vi "control loop output action.vi"(11 "control loop data in":T1) -> (3 "control loop data out":T1)   [LabVIEW 2013, in "main engine.lvlib"]
doc: "This VI calls the output method of any modules specified by flags set in 'engine schedule.module run flags'. It also exchanges the data necessary for that method with the data in the engine tag bus. Any errors that occur are stored to be handled at the end of the engine's execution.\n\nSynchronous calls are handled inline. Asynchronous calls use a FIFO to communicate with a separate process launched during the initialization process."
uses:
  main engine.lvlib
  control loop data.ctl
  <vilib>/NI/Tag Bus/table/data table.ctl
  engine run schedule.ctl
  engine decimation schedule.ctl
  full module data.ctl
  <vilib>/NI/Tag Bus Module Framework/runtime/TBM module execution interface.lvclass
  module run state.ctl
  async executor/asynchronous executor reference.ctl
  async executor/async message to executor.ctl
  Runtime/async command notification.ctl
  Runtime/async error info.ctl
  <vilib>/NI/Tag Bus Module Framework/runtime/error classification.ctl
  <vilib>/NI/Tag Bus Module Framework/module configuration/TBM module configuration.lvclass
  module method data.ctl
  <vilib>/NI/Tag Bus/table/transfer specification.ctl
  <vilib>/NI/Tag Bus/tag/Data Type.ctl
  fault handling spec.ctl
  Configuration/Error Actions.ctl
  <vilib>/NI/Tag Bus/table/data table.lvlib
  <vilib>/NI/Tag Bus/tag/tag descriptor.lvclass
  Configuration/Standard Engine Configuration.lvclass
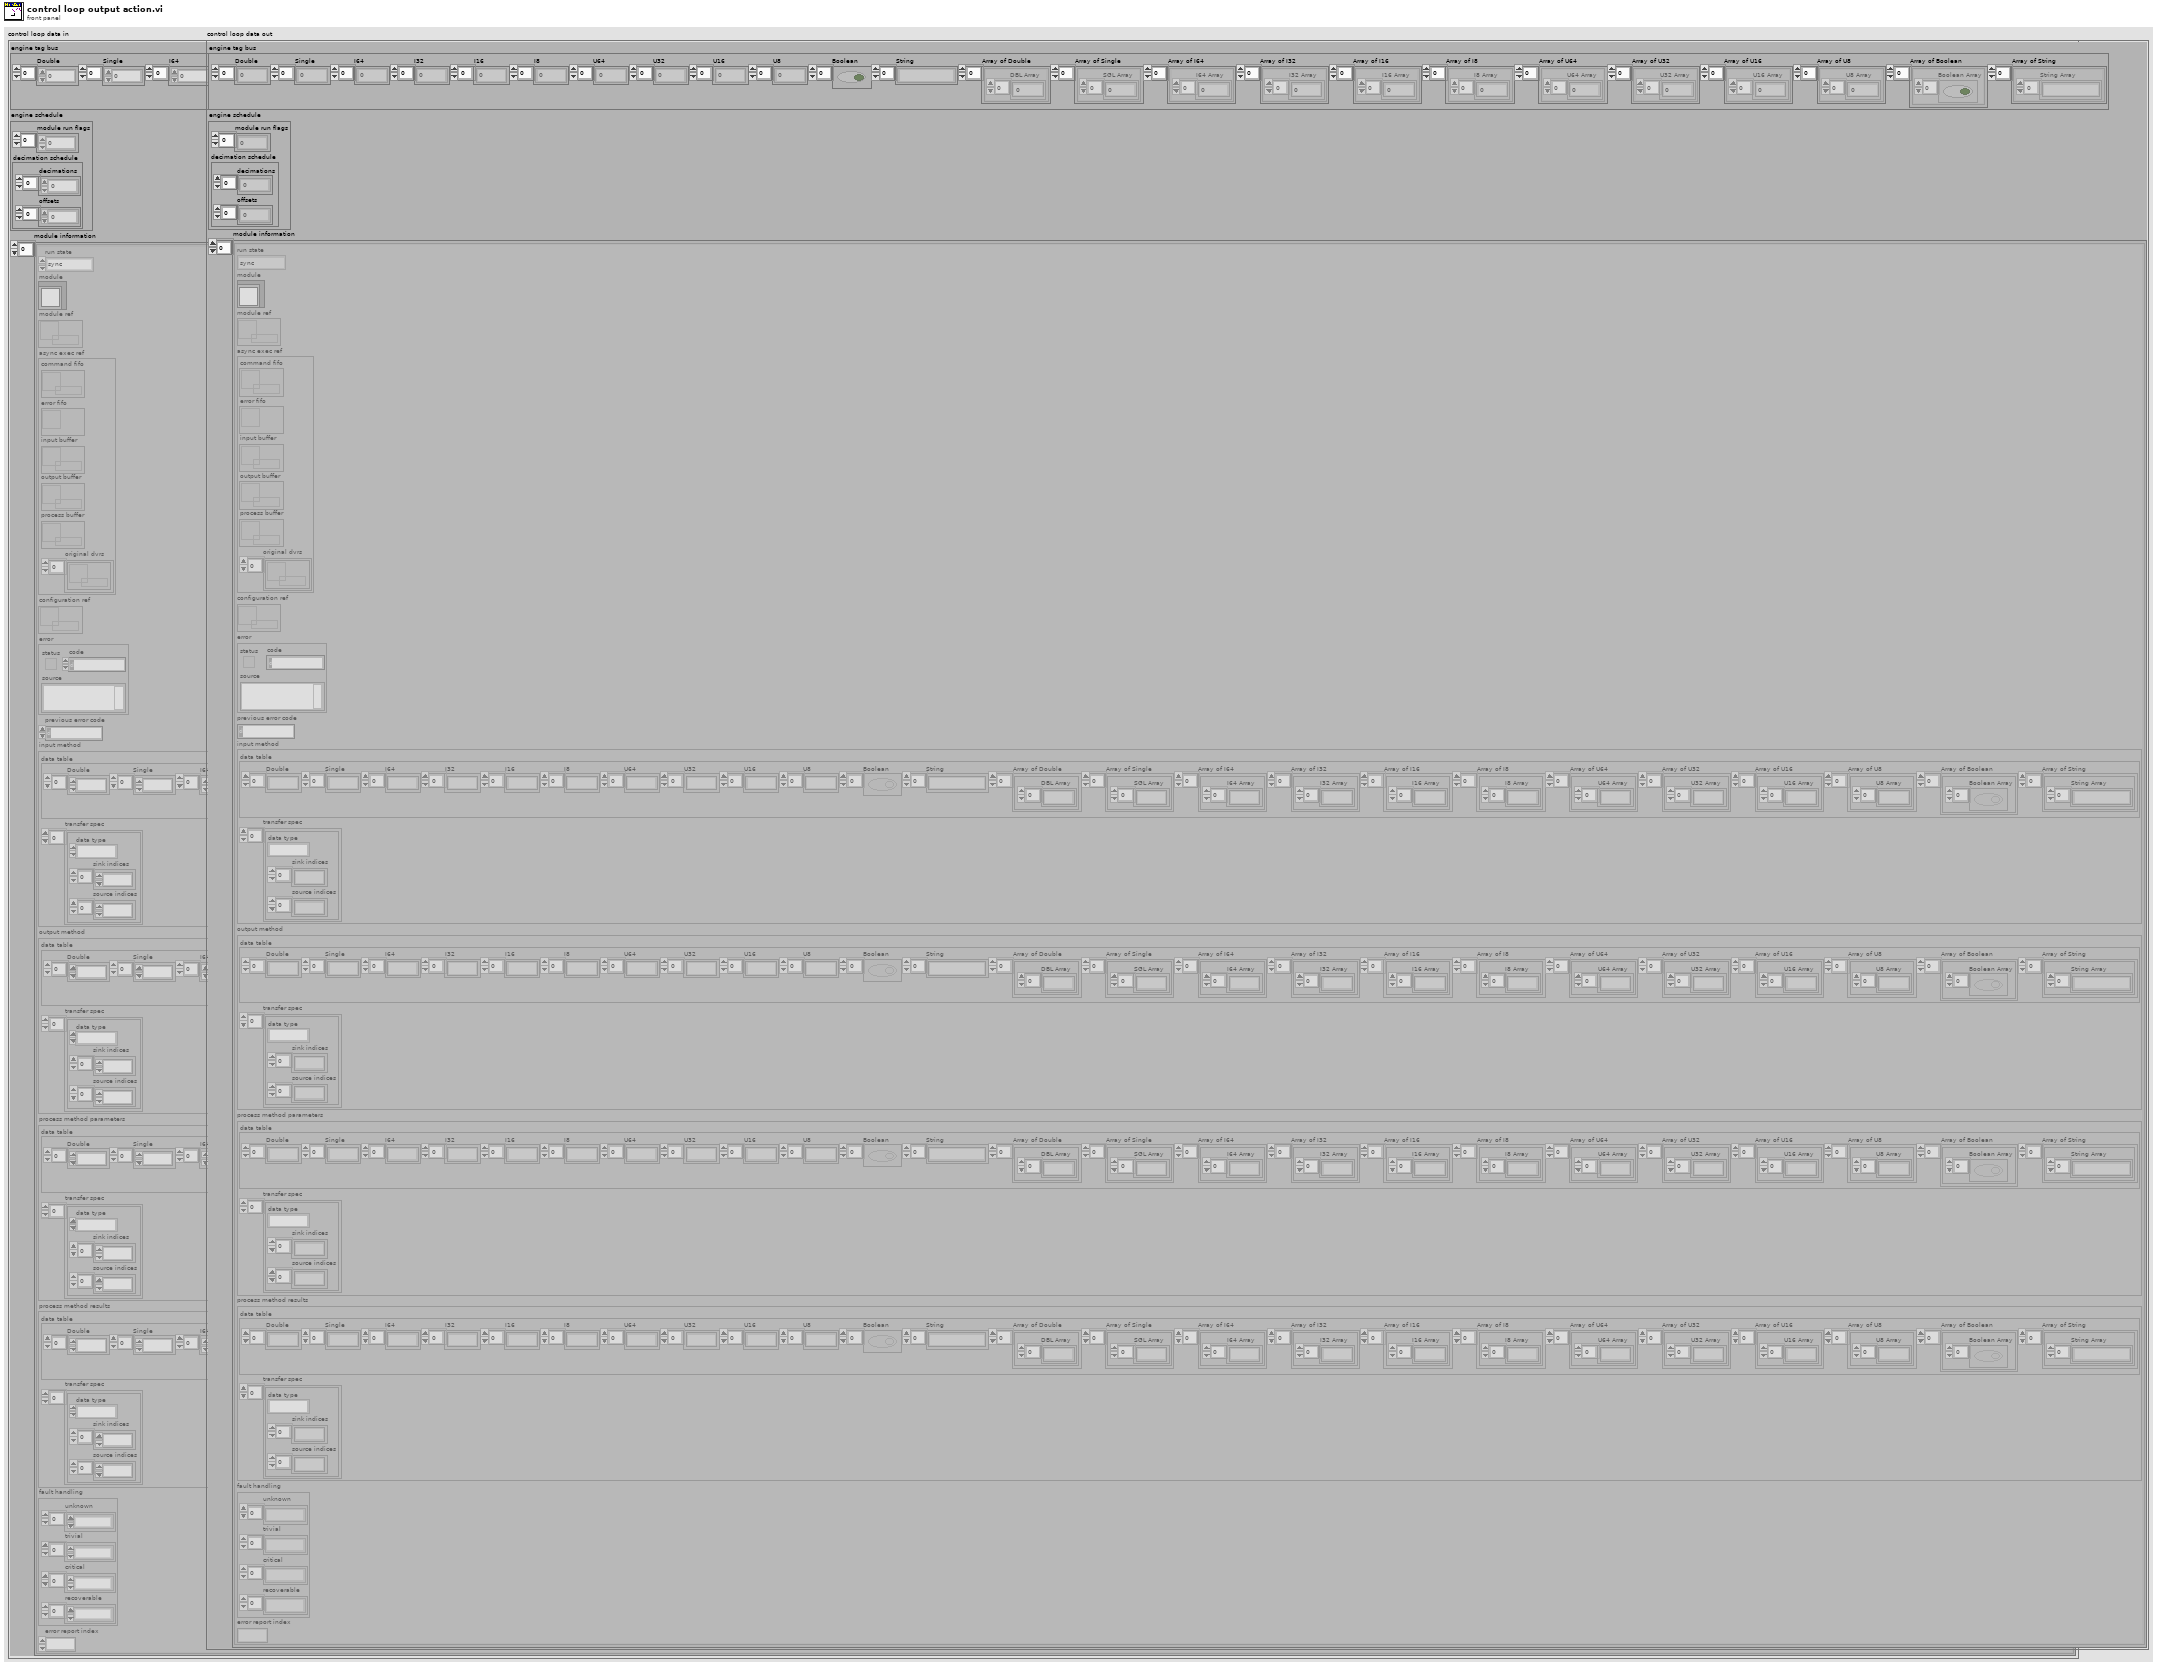
[diagram p1: front panel]
types:
  T1 = typedef "main engine.lvlib/control loop data.ctl" = cluster{"engine tag bus":T2, "engine schedule":T3, "module information":T5[]}
  T2 = typedef "tag bus.lvlib/data table.lvlib/data table.ctl" = cluster{"Double":dbl[], "Single":sgl[], "I64":i64[], "I32":i32[], "I16":i16[], "I8":i8[], "U64":u64[], "U32":u32[], "U16":u16[], "U8":u8[], "Boolean":bool[], "String":string[], "Array of Double":cluster{"DBL Array":dbl[]}[], "Array of Single":cluster{"SGL Array":sgl[]}[], "Array of I64":cluster{"I64 Array":i64[]}[], "Array of I32":cluster{"I32 Array":i32[]}[], "Array of I16":cluster{"I16 Array":i16[]}[], "Array of I8":cluster{"I8 Array":i8[]}[], "Array of U64":cluster{"U64 Array":u64[]}[], "Array of U32":cluster{"U32 Array":u32[]}[], "Array of U16":cluster{"U16 Array":u16[]}[], "Array of U8":cluster{"U8 Array":u8[]}[], "Array of Boolean":cluster{"Boolean Array":bool[]}[], "Array of String":cluster{"String Array":string[]}[]}
  T3 = typedef "main engine.lvlib/engine run schedule.ctl" = cluster{"module run flags":u8[], "decimation schedule":T4}
  T4 = typedef "main engine.lvlib/engine decimation schedule.ctl" = cluster{"decimations":u16[], "offsets":u16[]}
  T5 = typedef "main engine.lvlib/full module data.ctl" = cluster{"run state":T6, "module":refnum<class "TBM module execution interface.lvclass">, "module ref":refnum<data-value>, "async exec ref":T7, "configuration ref":refnum<data-value>, "error":errorcluster, "previous error code":i32, "input method":T8, "output method":T8, "process method parameters":T8, "process method results":T8, "fault handling":T11, "error report index ":i32}
  T6 = typedef "main engine.lvlib/module run state.ctl" = enum16{"sync", "async"}
  T7 = typedef "main engine.lvlib/asynchronous executor reference.ctl" = cluster{"command fifo":refnum<k33>, "error fifo":refnum<k33>, "input buffer":refnum<k33>, "output buffer":refnum<k33>, "process buffer":refnum<k33>, "original dvrs":refnum<data-value>[]}
  T8 = typedef "main engine.lvlib/module method data.ctl" = cluster{"data table":T2, "transfer spec":T9[]}
  T9 = typedef "tag bus.lvlib/data table.lvlib/transfer specification.ctl" = cluster{"data type":T10, "sink indices":i32[], "source indices":i32[]}
  T10 = typedef "tag bus.lvlib/tag descriptor.lvclass/Data Type.ctl" = enum16{"Double", "Single", "I64", "I32", "I16", "I8", "U64", "U32", "U16", "U8", "Boolean", "String", "Array of Double", "Array of Single", "Array of I64", "Array of I32", "Array of I16", "Array of I8", "Array of U64", "Array of U32", "Array of U16", "Array of U8", "Array of Boolean", "Array of String"}
  T11 = typedef "main engine.lvlib/fault handling spec.ctl" = cluster{"unknown":T12[], "trivial":T12[], "critical":T12[], "recoverable":T12[]}
  T12 = typedef "Standard Engine Configuration.lvclass/Error Actions.ctl" = enum16{"Clear", "Notify", "Log", "Stop Component", "Stop Engine", "Safe State", "Attempt Recovery"}
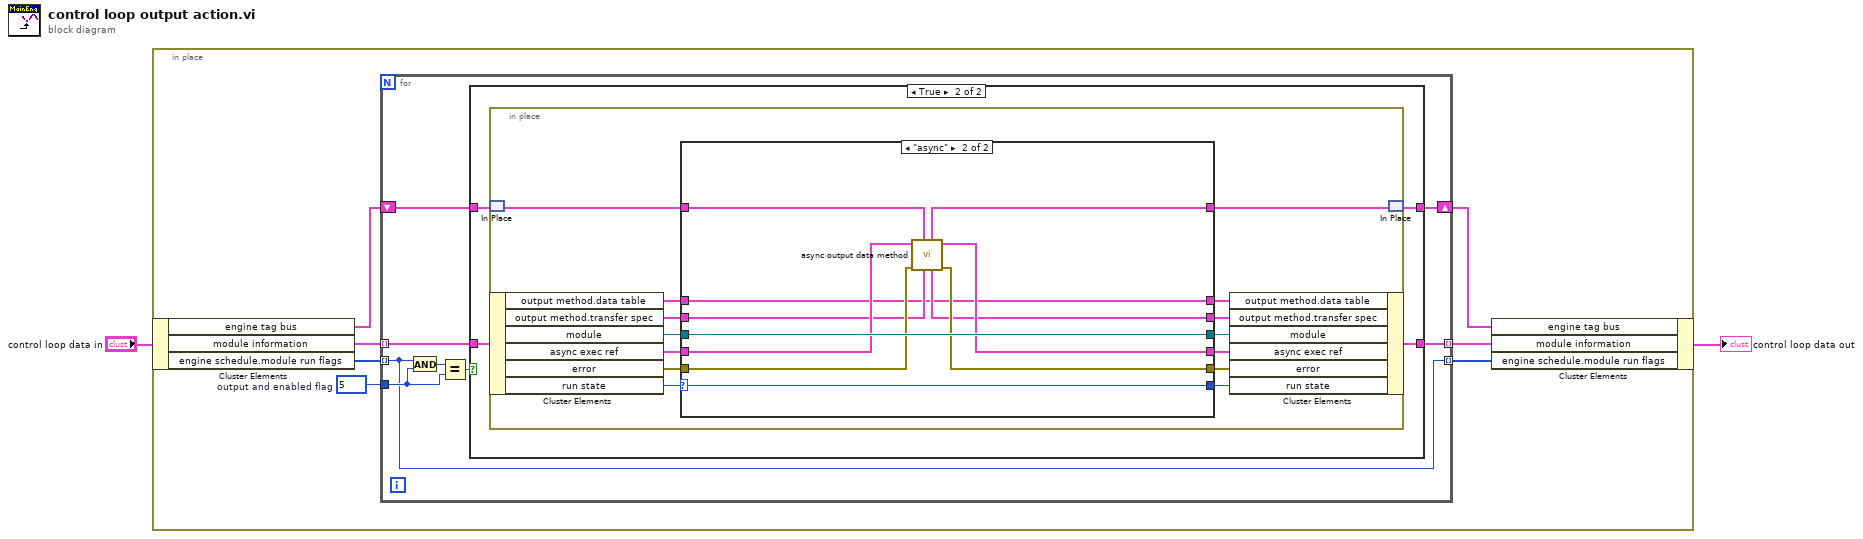
[diagram p0: block diagram]
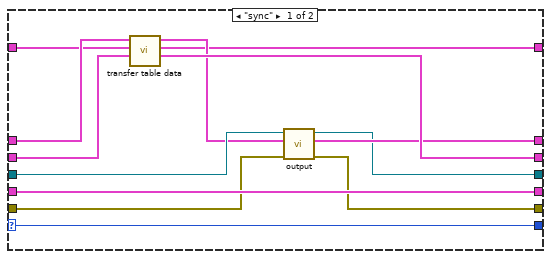
[diagram p3: hidden frame]
diagram:
  n1 = in-place {
    w4 = u8 5  # output and enabled flag
    n2 = in-place-cluster #1("control loop data in") -> ("engine tag bus"=w8:T2, "module information"=w6:T5[], "engine schedule.module run flags"=w9:u8[])
    n3 = for {
      tunnel: w9 -> [w10] mode=indexing
      shift-right: [w16] -> w7
      shift-left: w8 -> [w17]
      tunnel: w6 -> [w15] mode=indexing
      tunnel: [w14] -> w5 mode=indexing
      tunnel: w4 -> [w12]
      tunnel: [w10] -> w3 mode=indexing
      n4 = And(x=w10, y=w12) -> (x .and. y?=w13:u8)
      n5 = Equal?(x=w13, y=w12) -> (x = y?=w11:bool)
      n6 = case shown="True" w11 {
        tunnel: w17 -> [w19 w23]
        tunnel: [w19 w22] -> w16
        tunnel: w15 -> [w18 w21]
        tunnel: [w18 w20] -> w14
        frame False {
        }
        frame True {
          n7 = in-place {
            n8 = in-place-match #2(w23) -> (w35:T2)
            n9 = in-place-cluster #3(w21) -> ("output method.data table"=w26:T2, "output method.transfer spec"=w34:T9[], "module"=w33:refnum<class "TBM module execution interface.lvclass">, "async exec ref"=w30:T7, "error"=w29:errorcluster, "run state"=w37:T6)
            n10 = case shown="\"async\"" w37 {
              selector: w37 -> [w49 w61]
              tunnel: [w38 w58] -> w36
              tunnel: w35 -> [w40 w59]
              tunnel: w34 -> [w47 w53]
              tunnel: w33 -> [w43 w60]
              tunnel: [w42 w60] -> w32
              tunnel: [w50 w56] -> w31
              tunnel: w30 -> [w50 w55]
              tunnel: w29 -> [w46 w54]
              tunnel: [w49 w61] -> w28
              tunnel: [w48 w52] -> w27
              tunnel: w26 -> [w41 w51]
              tunnel: [w45 w57] -> w25
              tunnel: [w44 w51] -> w24
              frame "sync" {
                n11 = call <vilib>:"transfer table data.vi"("transfer specification in"=w47, "data table source in"=w40, "data table sink in"=w41) -> ("transfer specification out"=w48:T9[], "data table source out"=w38:T2, "data table sink out"=w39:T2)  [unwired: 6 in]
                n12 = call-dynamic "output.vi"("error in"=w46, "output data"=w39, "module in"=w43) -> ("error out"=w45:errorcluster, "output allocation"=w44:T2, "module out"=w42:refnum<class "TBM module execution interface.lvclass">)  [unwired: 6 in]
              }
              frame "async" {
                n13 = call "async output data method.vi"("transfer specification in"=w53, "engine tag data in"=w59, "error in"=w54, "async exec in"=w55) -> ("error out"=w57:errorcluster, "async exec out"=w56:T7, "transfer specification out"=w52:T9[], "engine tag data out"=w58:T2)  [unwired: 4 in]
              }
            }
            n14 = in-place-cluster #3("output method.data table"=w24, "output method.transfer spec"=w27, "module"=w32, "async exec ref"=w31, "error"=w25, "run state"=w28) -> (w20:T5)
            n15 = in-place-match #2(w36) -> (w22:T2)
          }
        }
      }
    }
    n16 = in-place-cluster #1("engine tag bus"=w7, "module information"=w5, "engine schedule.module run flags"=w3) -> (→"control loop data out":T1)
  }
